vi "App - analyze RUS V6.vi"() -> ()   [LabVIEW 2015] (continued)
, "file path"=path "D:/Data/Ultrasound/LSCO/LSCO22__130814c/5_Cooling_2nd_try/September_2014/091714/50.16200K_500_2500_2.10000V_0.00000T_Sep17-2014__11-53-36_001_091714.bin", "last mod"=timestamp(3493814016 s since 1904-01-01), "file name str"="D:\\Data\\Ultrasound\\LSCO\\LSCO22__130814c\\5_Cooling_2nd_try\\September_2014\\091714\\50.16200K_500_2500_2.10000V_0.00000T_Sep17-2014__11-53-36_001_091714.bin", "mod time(min)"=58230233.6, "file format"=enum."binary", "power(V)"=2.1, "Magn Field(T) "=0.0}, {"temperature"=50.094, "temperature str"="50.09400", "file path"=path "D:/Data/Ultrasound/LSCO/LSCO22__130814c/5_Cooling_2nd_try/September_2014/091714/50.09400K_500_2500_2.10000V_0.00000T_Sep17-2014__11-54-56_001_091714.bin", "last mod"=timestamp(3493814096 s since 1904-01-01), "file name str"="D:\\Data\\Ultrasound\\LSCO\\LSCO22__130814c\\5_Cooling_2nd_try\\September_2014\\091714\\50.09400K_500_2500_2.10000V_0.00000T_Sep17-2014__11-54-56_001_091714.bin", "mod time(min)"=58230234.93333333, "file format"=enum."binary", "power(V)"=2.1, "Magn Field(T) "=0.0}, {"temperature"=50.029, "temperature str"="50.02900", "file path"=path "D:/Data/Ultrasound/LSCO/LSCO22__130814c/5_Cooling_2nd_try/September_2014/091714/50.02900K_500_2500_2.10000V_0.00000T_Sep17-2014__11-56-15_001_091714.bin", "last mod"=timestamp(3493814175 s since 1904-01-01), "file name str"="D:\\Data\\Ultrasound\\LSCO\\LSCO22__130814c\\5_Cooling_2nd_try\\September_2014\\091714\\50.02900K_500_2500_2.10000V_0.00000T_Sep17-2014__11-56-15_001_091714.bin", "mod time(min)"=58230236.25, "file format"=enum."binary", "power(V)"=2.1, "Magn Field(T) "=0.0}, {"temperature"=49.955, "temperature str"="49.95500", "file path"=path "D:/Data/Ultrasound/LSCO/LSCO22__130814c/5_Cooling_2nd_try/September_2014/091714/49.95500K_500_2500_2.10000V_0.00000T_Sep17-2014__11-57-34_001_091714.bin", "last mod"=timestamp(3493814254 s since 1904-01-01), "file name str"="D:\\Data\\Ultrasound\\LSCO\\LSCO22__130814c\\5_Cooling_2nd_try\\September_2014\\091714\\49.95500K_500_2500_2.10000V_0.00000T_Sep17-2014__11-57-34_001_091714.bin", "mod time(min)"=58230237.56666667, "file format"=enum."binary", "power(V)"=2.1, "Magn Field(T) "=0.0}, {"temperature"=49.895, "temperature str"="49.89500", "file path"=path "D:/Data/Ultrasound/LSCO/LSCO22__130814c/5_Cooling_2nd_try/September_2014/091714/49.89500K_500_2500_2.10000V_0.00000T_Sep17-2014__11-58-54_001_091714.bin", "last mod"=timestamp(3493814334 s since 1904-01-01), "file name str"="D:\\Data\\Ultrasound\\LSCO\\LSCO22__130814c\\5_Cooling_2nd_try\\September_2014\\091714\\49.89500K_500_2500_2.10000V_0.00000T_Sep17-2014__11-58-54_001_091714.bin", "mod time(min)"=58230238.9, "file format"=enum."binary", "power(V)"=2.1, "Magn Field(T) "=0.0}, {"temperature"=49.828, "temperature str"="49.82800", "file path"=path "D:/Data/Ultrasound/LSCO/LSCO22__130814c/5_Cooling_2nd_try/September_2014/091714/49.82800K_500_2500_2.10000V_0.00000T_Sep17-2014__12-00-13_001_091714.bin", "last mod"=timestamp(3493814413 s since 1904-01-01), "file name str"="D:\\Data\\Ultrasound\\LSCO\\LSCO22__130814c\\5_Cooling_2nd_try\\September_2014\\091714\\49.82800K_500_2500_2.10000V_0.00000T_Sep17-2014__12-00-13_001_091714.bin", "mod time(min)"=58230240.21666667, "file format"=enum."binary", "power(V)"=2.1, "Magn Field(T) "=0.0}, {"temperature"=49.758, "temperature str"="49.75800", "file path"=path "D:/Data/Ultrasound/LSCO/LSCO22__130814c/5_Cooling_2nd_try/September_2014/091714/49.75800K_500_2500_2.10000V_0.00000T_Sep17-2014__12-01-32_001_091714.bin", "last mod"=timestamp(3493814492 s since 1904-01-01), "file name str"="D:\\Data\\Ultrasound\\LSCO\\LSCO22__130814c\\5_Cooling_2nd_try\\September_2014\\091714\\49.75800K_500_2500_2.10000V_0.00000T_Sep17-2014__12-01-32_001_091714.bin", "mod time(min)"=58230241.53333333, "file format"=enum."binary", "power(V)"=2.1, "Magn Field(T) "=0.0}, {"temperature"=49.694, "temperature str"="49.69400", "file path"=path "D:/Data/Ultrasound/LSCO/LSCO22__130814c/5_Cooling_2nd_try/September_2014/091714/49.69400K_500_2500_2.10000V_0.00000T_Sep17-2014__12-02-52_001_091714.bin", "last mod"=timestamp(3493814572 s since 1904-01-01), "file name str"="D:\\Data\\Ultrasound\\LSCO\\LSCO22__130814c\\5_Cooling_2nd_try\\September_2014\\091714\\49.69400K_500_2500_2.10000V_0.00000T_Sep17-2014__12-02-52_001_091714.bin", "mod time(min)"=58230242.86666667, "file format"=enum."binary", "power(V)"=2.1, "Magn Field(T) "=0.0}, {"temperature"=49.627, "temperature str"="49.62700", "file path"=path "D:/Data/Ultrasound/LSCO/LSCO22__130814c/5_Cooling_2nd_try/September_2014/091714/49.62700K_500_2500_2.10000V_0.00000T_Sep17-2014__12-04-11_001_091714.bin", "last mod"=timestamp(3493814651 s since 1904-01-01), "file name str"="D:\\Data\\Ultrasound\\LSCO\\LSCO22__130814c\\5_Cooling_2nd_try\\September_2014\\091714\\49.62700K_500_2500_2.10000V_0.00000T_Sep17-2014__12-04-11_001_091714.bin", "mod time(min)"=58230244.18333333, "file format"=enum."binary", "power(V)"=2.1, "Magn Field(T) "=0.0}, {"temperature"=49.555, "temperature str"="49.55500", "file path"=path "D:/Data/Ultrasound/LSCO/LSCO22__130814c/5_Cooling_2nd_try/September_2014/091714/49.55500K_500_2500_2.10000V_0.00000T_Sep17-2014__12-05-31_001_091714.bin", "last mod"=timestamp(3493814731 s since 1904-01-01), "file name str"="D:\\Data\\Ultrasound\\LSCO\\LSCO22__130814c\\5_Cooling_2nd_try\\September_2014\\091714\\49.55500K_500_2500_2.10000V_0.00000T_Sep17-2014__12-05-31_001_091714.bin", "mod time(min)"=58230245.516666666, "file format"=enum."binary", "power(V)"=2.1, "Magn Field(T) "=0.0}, {"temperature"=49.488, "temperature str"="49.48800", "file path"=path "D:/Data/Ultrasound/LSCO/LSCO22__130814c/5_Cooling_2nd_try/September_2014/091714/49.48800K_500_2500_2.10000V_0.00000T_Sep17-2014__12-06-50_001_091714.bin", "last mod"=timestamp(3493814810 s since 1904-01-01), "file name str"="D:\\Data\\Ultrasound\\LSCO\\LSCO22__130814c\\5_Cooling_2nd_try\\September_2014\\091714\\49.48800K_500_2500_2.10000V_0.00000T_Sep17-2014__12-06-50_001_091714.bin", "mod time(min)"=58230246.833333336, "file format"=enum."binary", "power(V)"=2.1, "Magn Field(T) "=0.0}, {"temperature"=49.42, "temperature str"="49.42000", "file path"=path "D:/Data/Ultrasound/LSCO/LSCO22__130814c/5_Cooling_2nd_try/September_2014/091714/49.42000K_500_2500_2.10000V_0.00000T_Sep17-2014__12-08-09_001_091714.bin", "last mod"=timestamp(3493814889 s since 1904-01-01), "file name str"="D:\\Data\\Ultrasound\\LSCO\\LSCO22__130814c\\5_Cooling_2nd_try\\September_2014\\091714\\49.42000K_500_2500_2.10000V_0.00000T_Sep17-2014__12-08-09_001_091714.bin", "mod time(min)"=58230248.15, "file format"=enum."binary", "power(V)"=2.1, "Magn Field(T) "=0.0}, {"temperature"=49.351, "temperature str"="49.35100", "file path"=path "D:/Data/Ultrasound/LSCO/LSCO22__130814c/5_Cooling_2nd_try/September_2014/091714/49.35100K_500_2500_2.10000V_0.00000T_Sep17-2014__12-09-29_001_091714.bin", "last mod"=timestamp(3493814969 s since 1904-01-01), "file name str"="D:\\Data\\Ultrasound\\LSCO\\LSCO22__130814c\\5_Cooling_2nd_try\\September_2014\\091714\\49.35100K_500_2500_2.10000V_0.00000T_Sep17-2014__12-09-29_001_091714.bin", "mod time(min)"=58230249.483333334, "file format"=enum."binary", "power(V)"=2.1, "Magn Field(T) "=0.0}, {"temperature"=49.284, "temperature str"="49.28400", "file path"=path "D:/Data/Ultrasound/LSCO/LSCO22__130814c/5_Cooling_2nd_try/September_2014/091714/49.28400K_500_2500_2.10000V_0.00000T_Sep17-2014__12-10-48_001_091714.bin", "last mod"=timestamp(3493815048 s since 1904-01-01), "file name str"="D:\\Data\\Ultrasound\\LSCO\\LSCO22__130814c\\5_Cooling_2nd_try\\September_2014\\091714\\49.28400K_500_2500_2.10000V_0.00000T_Sep17-2014__12-10-48_001_091714.bin", "mod time(min)"=58230250.8, "file format"=enum."binary", "power(V)"=2.1, "Magn Field(T) "=0.0}, {"temperature"=49.214, "temperature str"="49.21400", "file path"=path "D:/Data/Ultrasound/LSCO/LSCO22__130814c/5_Cooling_2nd_try/September_2014/091714/49.21400K_500_2500_2.10000V_0.00000T_Sep17-2014__12-12-07_001_091714.bin", "last mod"=timestamp(3493815127 s since 1904-01-01), "file name str"="D:\\Data\\Ultrasound\\LSCO\\LSCO22__130814c\\5_Cooling_2nd_try\\September_2014\\091714\\49.21400K_500_2500_2.10000V_0.00000T_Sep17-2014__12-12-07_001_091714.bin", "mod time(min)"=58230252.11666667, "file format"=enum."binary", "power(V)"=2.1, "Magn Field(T) "=0.0}, {"temperature"=49.15, "temperature str"="49.15000", "file path"=path "D:/Data/Ultrasound/LSCO/LSCO22__130814c/5_Cooling_2nd_try/September_2014/091714/49.15000K_500_2500_2.10000V_0.00000T_Sep17-2014__12-13-27_001_091714.bin", "last mod"=timestamp(3493815207 s since 1904-01-01), "file name str"="D:\\Data\\Ultrasound\\LSCO\\LSCO22__130814c\\5_Cooling_2nd_try\\September_2014\\091714\\49.15000K_500_2500_2.10000V_0.00000T_Sep17-2014__12-13-27_001_091714.bin", "mod time(min)"=58230253.45, "file format"=enum."binary", "power(V)"=2.1, "Magn Field(T) "=0.0}, {"temperature"=49.077, "temperature str"="49.07700", "file path"=path "D:/Data/Ultrasound/LSCO/LSCO22__130814c/5_Cooling_2nd_try/September_2014/091714/49.07700K_500_2500_2.10000V_0.00000T_Sep17-2014__12-14-46_001_091714.bin", "last mod"=timestamp(3493815286 s since 1904-01-01), "file name str"="D:\\Data\\Ultrasound\\LSCO\\LSCO22__130814c\\5_Cooling_2nd_try\\September_2014\\091714\\49.07700K_500_2500_2.10000V_0.00000T_Sep17-2014__12-14-46_001_091714.bin", "mod time(min)"=58230254.766666666, "file format"=enum."binary", "power(V)"=2.1, "Magn Field(T) "=0.0}, {"temperature"=49.008, "temperature str"="49.00800", "file path"=path "D:/Data/Ultrasound/LSCO/LSCO22__130814c/5_Cooling_2nd_try/September_2014/091714/49.00800K_500_2500_2.10000V_0.00000T_Sep17-2014__12-16-06_001_091714.bin", "last mod"=timestamp(3493815366 s since 1904-01-01), "file name str"="D:\\Data\\Ultrasound\\LSCO\\LSCO22__130814c\\5_Cooling_2nd_try\\September_2014\\091714\\49.00800K_500_2500_2.10000V_0.00000T_Sep17-2014__12-16-06_001_091714.bin", "mod time(min)"=58230256.1, "file format"=enum."binary", "power(V)"=2.1, "Magn Field(T) "=0.0}, {"temperature"=48.942, "temperature str"="48.94200", "file path"=path "D:/Data/Ultrasound/LSCO/LSCO22__130814c/5_Cooling_2nd_try/September_2014/091714/48.94200K_500_2500_2.10000V_0.00000T_Sep17-2014__12-17-25_001_091714.bin", "last mod"=timestamp(3493815445 s since 1904-01-01), "file name str"="D:\\Data\\Ultrasound\\LSCO\\LSCO22__130814c\\5_Cooling_2nd_try\\September_2014\\091714\\48.94200K_500_2500_2.10000V_0.00000T_Sep17-2014__12-17-25_001_091714.bin", "mod time(min)"=58230257.416666664, "file format"=enum."binary", "power(V)"=2.1, "Magn Field(T) "=0.0}, {"temperature"=48.873, "temperature str"="48.87300", "file path"=path "D:/Data/Ultrasound/LSCO/LSCO22__130814c/5_Cooling_2nd_try/September_2014/091714/48.87300K_500_2500_2.10000V_0.00000T_Sep17-2014__12-18-44_001_091714.bin", "last mod"=timestamp(3493815524 s since 1904-01-01), "file name str"="D:\\Data\\Ultrasound\\LSCO\\LSCO22__130814c\\5_Cooling_2nd_try\\September_2014\\091714\\48.87300K_500_2500_2.10000V_0.00000T_Sep17-2014__12-18-44_001_091714.bin", "mod time(min)"=58230258.733333334, "file format"=enum."binary", "power(V)"=2.1, "Magn Field(T) "=0.0}, {"temperature"=48.805, "temperature str"="48.80500", "file path"=path "D:/Data/Ultrasound/LSCO/LSCO22__130814c/5_Cooling_2nd_try/September_2014/091714/48.80500K_500_2500_2.10000V_0.00000T_Sep17-2014__12-20-04_001_091714.bin", "last mod"=timestamp(3493815604 s since 1904-01-01), "file name str"="D:\\Data\\Ultrasound\\LSCO\\LSCO22__130814c\\5_Cooling_2nd_try\\September_2014\\091714\\48.80500K_500_2500_2.10000V_0.00000T_Sep17-2014__12-20-04_001_091714.bin", "mod time(min)"=58230260.06666667, "file format"=enum."binary", "power(V)"=2.1, "Magn Field(T) "=0.0}, {"temperature"=48.734, "temperature str"="48.73400", "file path"=path "D:/Data/Ultrasound/LSCO/LSCO22__130814c/5_Cooling_2nd_try/September_2014/091714/48.73400K_500_2500_2.10000V_0.00000T_Sep17-2014__12-21-23_001_091714.bin", "last mod"=timestamp(3493815683 s since 1904-01-01), "file name str"="D:\\Data\\Ultrasound\\LSCO\\LSCO22__130814c\\5_Cooling_2nd_try\\September_2014\\091714\\48.73400K_500_2500_2.10000V_0.00000T_Sep17-2014__12-21-23_001_091714.bin", "mod time(min)"=58230261.38333333, "file format"=enum."binary", "power(V)"=2.1, "Magn Field(T) "=0.0}, {"temperature"=48.668, "temperature str"="48.66800", "file path"=path "D:/Data/Ultrasound/LSCO/LSCO22__130814c/5_Cooling_2nd_try/September_2014/091714/48.66800K_500_2500_2.10000V_0.00000T_Sep17-2014__12-22-42_001_091714.bin", "last mod"=timestamp(3493815762 s since 1904-01-01), "file name str"="D:\\Data\\Ultrasound\\LSCO\\LSCO22__130814c\\5_Cooling_2nd_try\\September_2014\\091714\\48.66800K_500_2500_2.10000V_0.00000T_Sep17-2014__12-22-42_001_091714.bin", "mod time(min)"=58230262.7, "file format"=enum."binary", "power(V)"=2.1, "Magn Field(T) "=0.0}, {"temperature"=48.596, "temperature str"="48.59600", "file path"=path "D:/Data/Ultrasound/LSCO/LSCO22__130814c/5_Cooling_2nd_try/September_2014/091714/48.59600K_500_2500_2.10000V_0.00000T_Sep17-2014__12-24-02_001_091714.bin", "last mod"=timestamp(3493815842 s since 1904-01-01), "file name str"="D:\\Data\\Ultrasound\\LSCO\\LSCO22__130814c\\5_Cooling_2nd_try\\September_2014\\091714\\48.59600K_500_2500_2.10000V_0.00000T_Sep17-2014__12-24-02_001_091714.bin", "mod time(min)"=58230264.03333333, "file format"=enum."binary", "power(V)"=2.1, "Magn Field(T) "=0.0}, {"temperature"=48.529, "temperature str"="48.52900", "file path"=path "D:/Data/Ultrasound/LSCO/LSCO22__130814c/5_Cooling_2nd_try/September_2014/091714/48.52900K_500_2500_2.10000V_0.00000T_Sep17-2014__12-25-21_001_091714.bin", "last mod"=timestamp(3493815921 s since 1904-01-01), "file name str"="D:\\Data\\Ultrasound\\LSCO\\LSCO22__130814c\\5_Cooling_2nd_try\\September_2014\\091714\\48.52900K_500_2500_2.10000V_0.00000T_Sep17-2014__12-25-21_001_091714.bin", "mod time(min)"=58230265.35, "file format"=enum."binary", "power(V)"=2.1, "Magn Field(T) "=0.0}, {"temperature"=48.459, "temperature str"="48.45900", "file path"=path "D:/Data/Ultrasound/LSCO/LSCO22__130814c/5_Cooling_2nd_try/September_2014/091714/48.45900K_500_2500_2.10000V_0.00000T_Sep17-2014__12-26-41_001_091714.bin", "last mod"=timestamp(3493816001 s since 1904-01-01), "file name str"="D:\\Data\\Ultrasound\\LSCO\\LSCO22__130814c\\5_Cooling_2nd_try\\September_2014\\091714\\48.45900K_500_2500_2.10000V_0.00000T_Sep17-2014__12-26-41_001_091714.bin", "mod time(min)"=58230266.68333333, "file format"=enum."binary", "power(V)"=2.1, "Magn Field(T) "=0.0}, {"temperature"=48.393, "temperature str"="48.39300", "file path"=path "D:/Data/Ultrasound/LSCO/LSCO22__130814c/5_Cooling_2nd_try/September_2014/091714/48.39300K_500_2500_2.10000V_0.00000T_Sep17-2014__12-28-00_001_091714.bin", "last mod"=timestamp(3493816080 s since 1904-01-01), "file name str"="D:\\Data\\Ultrasound\\LSCO\\LSCO22__130814c\\5_Cooling_2nd_try\\September_2014\\091714\\48.39300K_500_2500_2.10000V_0.00000T_Sep17-2014__12-28-00_001_091714.bin", "mod time(min)"=58230268.0, "file format"=enum."binary", "power(V)"=2.1, "Magn Field(T) "=0.0}, {"temperature"=48.325, "temperature str"="48.32500", "file path"=path "D:/Data/Ultrasound/LSCO/LSCO22__130814c/5_Cooling_2nd_try/September_2014/091714/48.32500K_500_2500_2.10000V_0.00000T_Sep17-2014__12-29-19_001_091714.bin", "last mod"=timestamp(3493816159 s since 1904-01-01), "file name str"="D:\\Data\\Ultrasound\\LSCO\\LSCO22__130814c\\5_Cooling_2nd_try\\September_2014\\091714\\48.32500K_500_2500_2.10000V_0.00000T_Sep17-2014__12-29-19_001_091714.bin", "mod time(min)"=58230269.31666667, "file format"=enum."binary", "power(V)"=2.1, "Magn Field(T) "=0.0}, {"temperature"=48.248, "temperature str"="48.24800", "file path"=path "D:/Data/Ultrasound/LSCO/LSCO22__130814c/5_Cooling_2nd_try/September_2014/091714/48.24800K_500_2500_2.10000V_0.00000T_Sep17-2014__12-30-39_001_091714.bin", "last mod"=timestamp(3493816239 s since 1904-01-01), "file name str"="D:\\Data\\Ultrasound\\LSCO\\LSCO22__130814c\\5_Cooling_2nd_try\\September_2014\\091714\\48.24800K_500_2500_2.10000V_0.00000T_Sep17-2014__12-30-39_001_091714.bin", "mod time(min)"=58230270.65, "file format"=enum."binary", "power(V)"=2.1, "Magn Field(T) "=0.0}, {"temperature"=48.181, "temperature str"="48.18100", "file path"=path "D:/Data/Ultrasound/LSCO/LSCO22__130814c/5_Cooling_2nd_try/September_2014/091714/48.18100K_500_2500_2.10000V_0.00000T_Sep17-2014__12-31-58_001_091714.bin", "last mod"=timestamp(3493816318 s since 1904-01-01), "file name str"="D:\\Data\\Ultrasound\\LSCO\\LSCO22__130814c\\5_Cooling_2nd_try\\September_2014\\091714\\48.18100K_500_2500_2.10000V_0.00000T_Sep17-2014__12-31-58_001_091714.bin", "mod time(min)"=58230271.96666667, "file format"=enum."binary", "power(V)"=2.1, "Magn Field(T) "=0.0}, {"temperature"=48.115, "temperature str"="48.11500", "file path"=path "D:/Data/Ultrasound/LSCO/LSCO22__130814c/5_Cooling_2nd_try/September_2014/091714/48.11500K_500_2500_2.10000V_0.00000T_Sep17-2014__12-33-17_001_091714.bin", "last mod"=timestamp(3493816397 s since 1904-01-01), "file name str"="D:\\Data\\Ultrasound\\LSCO\\LSCO22__130814c\\5_Cooling_2nd_try\\September_2014\\091714\\48.11500K_500_2500_2.10000V_0.00000T_Sep17-2014__12-33-17_001_091714.bin", "mod time(min)"=58230273.28333333, "file format"=enum."binary", "power(V)"=2.1, "Magn Field(T) "=0.0}, {"temperature"=48.042, "temperature str"="48.04200", "file path"=path "D:/Data/Ultrasound/LSCO/LSCO22__130814c/5_Cooling_2nd_try/September_2014/091714/48.04200K_500_2500_2.10000V_0.00000T_Sep17-2014__12-34-37_001_091714.bin", "last mod"=timestamp(3493816477 s since 1904-01-01), "file name str"="D:\\Data\\Ultrasound\\LSCO\\LSCO22__130814c\\5_Cooling_2nd_try\\September_2014\\091714\\48.04200K_500_2500_2.10000V_0.00000T_Sep17-2014__12-34-37_001_091714.bin", "mod time(min)"=58230274.61666667, "file format"=enum."binary", "power(V)"=2.1, "Magn Field(T) "=0.0}, {"temperature"=47.973, "temperature str"="47.97300", "file path"=path "D:/Data/Ultrasound/LSCO/LSCO22__130814c/5_Cooling_2nd_try/September_2014/091714/47.97300K_500_2500_2.10000V_0.00000T_Sep17-2014__12-35-56_001_091714.bin", "last mod"=timestamp(3493816556 s since 1904-01-01), "file name str"="D:\\Data\\Ultrasound\\LSCO\\LSCO22__130814c\\5_Cooling_2nd_try\\September_2014\\091714\\47.97300K_500_2500_2.10000V_0.00000T_Sep17-2014__12-35-56_001_091714.bin", "mod time(min)"=58230275.93333333, "file format"=enum."binary", "power(V)"=2.1, "Magn Field(T) "=0.0}, {"temperature"=47.908, "temperature str"="47.90800", "file path"=path "D:/Data/Ultrasound/LSCO/LSCO22__130814c/5_Cooling_2nd_try/September_2014/091714/47.90800K_500_2500_2.10000V_0.00000T_Sep17-2014__12-37-16_001_091714.bin", "last mod"=timestamp(3493816636 s since 1904-01-01), "file name str"="D:\\Data\\Ultrasound\\LSCO\\LSCO22__130814c\\5_Cooling_2nd_try\\September_2014\\091714\\47.90800K_500_2500_2.10000V_0.00000T_Sep17-2014__12-37-16_001_091714.bin", "mod time(min)"=58230277.266666666, "file format"=enum."binary", "power(V)"=2.1, "Magn Field(T) "=0.0}, {"temperature"=47.834, "temperature str"="47.83400", "file path"=path "D:/Data/Ultrasound/LSCO/LSCO22__130814c/5_Cooling_2nd_try/September_2014/091714/47.83400K_500_2500_2.10000V_0.00000T_Sep17-2014__12-38-35_001_091714.bin", "last mod"=timestamp(3493816715 s since 1904-01-01), "file name str"="D:\\Data\\Ultrasound\\LSCO\\LSCO22__130814c\\5_Cooling_2nd_try\\September_2014\\091714\\47.83400K_500_2500_2.10000V_0.00000T_Sep17-2014__12-38-35_001_091714.bin", "mod time(min)"=58230278.583333336, "file format"=enum."binary", "power(V)"=2.1, "Magn Field(T) "=0.0}, {"temperature"=47.764, "temperature str"="47.76400", "file path"=path "D:/Data/Ultrasound/LSCO/LSCO22__130814c/5_Cooling_2nd_try/September_2014/091714/47.76400K_500_2500_2.10000V_0.00000T_Sep17-2014__12-39-54_001_091714.bin", "last mod"=timestamp(3493816794 s since 1904-01-01), "file name str"="D:\\Data\\Ultrasound\\LSCO\\LSCO22__130814c\\5_Cooling_2nd_try\\September_2014\\091714\\47.76400K_500_2500_2.10000V_0.00000T_Sep17-2014__12-39-54_001_091714.bin", "mod time(min)"=58230279.9, "file format"=enum."binary", "power(V)"=2.1, "Magn Field(T) "=0.0}, {"temperature"=47.699, "temperature str"="47.69900", "file path"=path "D:/Data/Ultrasound/LSCO/LSCO22__130814c/5_Cooling_2nd_try/September_2014/091714/47.69900K_500_2500_2.10000V_0.00000T_Sep17-2014__12-41-14_001_091714.bin", "last mod"=timestamp(3493816874 s since 1904-01-01), "file name str"="D:\\Data\\Ultrasound\\LSCO\\LSCO22__130814c\\5_Cooling_2nd_try\\September_2014\\091714\\47.69900K_500_2500_2.10000V_0.00000T_Sep17-2014__12-41-14_001_091714.bin", "mod time(min)"=58230281.233333334, "file format"=enum."binary", "power(V)"=2.1, "Magn Field(T) "=0.0}, {"temperature"=47.625, "temperature str"="47.62500", "file path"=path "D:/Data/Ultrasound/LSCO/LSCO22__130814c/5_Cooling_2nd_try/September_2014/091714/47.62500K_500_2500_2.10000V_0.00000T_Sep17-2014__12-42-33_001_091714.bin", "last mod"=timestamp(3493816953 s since 1904-01-01), "file name str"="D:\\Data\\Ultrasound\\LSCO\\LSCO22__130814c\\5_Cooling_2nd_try\\September_2014\\091714\\47.62500K_500_2500_2.10000V_0.00000T_Sep17-2014__12-42-33_001_091714.bin", "mod time(min)"=58230282.55, "file format"=enum."binary", "power(V)"=2.1, "Magn Field(T) "=0.0}, {"temperature"=47.554, "temperature str"="47.55400", "file path"=path "D:/Data/Ultrasound/LSCO/LSCO22__130814c/5_Cooling_2nd_try/September_2014/091714/47.55400K_500_2500_2.10000V_0.00000T_Sep17-2014__12-43-52_001_091714.bin", "last mod"=timestamp(3493817032 s since 1904-01-01), "file name str"="D:\\Data\\Ultrasound\\LSCO\\LSCO22__130814c\\5_Cooling_2nd_try\\September_2014\\091714\\47.55400K_500_2500_2.10000V_0.00000T_Sep17-2014__12-43-52_001_091714.bin", "mod time(min)"=58230283.86666667, "file format"=enum."binary", "power(V)"=2.1, "Magn Field(T) "=0.0}, {"temperature"=47.487, "temperature str"="47.48700", "file path"=path "D:/Data/Ultrasound/LSCO/LSCO22__130814c/5_Cooling_2nd_try/September_2014/091714/47.48700K_500_2500_2.10000V_0.00000T_Sep17-2014__12-45-12_001_091714.bin", "last mod"=timestamp(3493817112 s since 1904-01-01), "file name str"="D:\\Data\\Ultrasound\\LSCO\\LSCO22__130814c\\5_Cooling_2nd_try\\September_2014\\091714\\47.48700K_500_2500_2.10000V_0.00000T_Sep17-2014__12-45-12_001_091714.bin", "mod time(min)"=58230285.2, "file format"=enum."binary", "power(V)"=2.1, "Magn Field(T) "=0.0}, {"temperature"=47.415, "temperature str"="47.41500", "file path"=path "D:/Data/Ultrasound/LSCO/LSCO22__130814c/5_Cooling_2nd_try/September_2014/091714/47.41500K_500_2500_2.10000V_0.00000T_Sep17-2014__12-46-31_001_091714.bin", "last mod"=timestamp(3493817191 s since 1904-01-01), "file name str"="D:\\Data\\Ultrasound\\LSCO\\LSCO22__130814c\\5_Cooling_2nd_try\\September_2014\\091714\\47.41500K_500_2500_2.10000V_0.00000T_Sep17-2014__12-46-31_001_091714.bin", "mod time(min)"=58230286.516666666, "file format"=enum."binary", "power(V)"=2.1, "Magn Field(T) "=0.0}, {"temperature"=47.343, "temperature str"="47.34300", "file path"=path "D:/Data/Ultrasound/LSCO/LSCO22__130814c/5_Cooling_2nd_try/September_2014/091714/47.34300K_500_2500_2.10000V_0.00000T_Sep17-2014__12-47-51_001_091714.bin", "last mod"=timestamp(3493817271 s since 1904-01-01), "file name str"="D:\\Data\\Ultrasound\\LSCO\\LSCO22__130814c\\5_Cooling_2nd_try\\September_2014\\091714\\47.34300K_500_2500_2.10000V_0.00000T_Sep17-2014__12-47-51_001_091714.bin", "mod time(min)"=58230287.85, "file format"=enum."binary", "power(V)"=2.1, "Magn Field(T) "=0.0}, {"temperature"=47.276, "temperature str"="47.27600", "file path"=path "D:/Data/Ultrasound/LSCO/LSCO22__130814c/5_Cooling_2nd_try/September_2014/091714/47.27600K_500_2500_2.10000V_0.00000T_Sep17-2014__12-49-10_001_091714.bin", "last mod"=timestamp(3493817350 s since 1904-01-01), "file name str"="D:\\Data\\Ultrasound\\LSCO\\LSCO22__130814c\\5_Cooling_2nd_try\\September_2014\\091714\\47.27600K_500_2500_2.10000V_0.00000T_Sep17-2014__12-49-10_001_091714.bin", "mod time(min)"=58230289.166666664, "file format"=enum."binary", "power(V)"=2.1, "Magn Field(T) "=0.0}, {"temperature"=47.203, "temperature str"="47.20300", "file path"=path "D:/Data/Ultrasound/LSCO/LSCO22__130814c/5_Cooling_2nd_try/September_2014/091714/47.20300K_500_2500_2.10000V_0.00000T_Sep17-2014__12-50-29_001_091714.bin", "last mod"=timestamp(3493817429 s since 1904-01-01), "file name str"="D:\\Data\\Ultrasound\\LSCO\\LSCO22__130814c\\5_Cooling_2nd_try\\September_2014\\091714\\47.20300K_500_2500_2.10000V_0.00000T_Sep17-2014__12-50-29_001_091714.bin", "mod time(min)"=58230290.483333334, "file format"=enum."binary", "power(V)"=2.1, "Magn Field(T) "=0.0}, {"temperature"=47.135, "temperature str"="47.13500", "file path"=path "D:/Data/Ultrasound/LSCO/LSCO22__130814c/5_Cooling_2nd_try/September_2014/091714/47.13500K_500_2500_2.10000V_0.00000T_Sep17-2014__12-51-49_001_091714.bin", "last mod"=timestamp(3493817509 s since 1904-01-01), "file name str"="D:\\Data\\Ultrasound\\LSCO\\LSCO22__130814c\\5_Cooling_2nd_try\\September_2014\\091714\\47.13500K_500_2500_2.10000V_0.00000T_Sep17-2014__12-51-49_001_091714.bin", "mod time(min)"=58230291.81666667, "file format"=enum."binary", "power(V)"=2.1, "Magn Field(T) "=0.0}, {"temperature"=47.061, "temperature str"="47.06100", "file path"=path "D:/Data/Ultrasound/LSCO/LSCO22__130814c/5_Cooling_2nd_try/September_2014/091714/47.06100K_500_2500_2.10000V_0.00000T_Sep17-2014__12-53-08_001_091714.bin", "last mod"=timestamp(3493817588 s since 1904-01-01), "file name str"="D:\\Data\\Ultrasound\\LSCO\\LSCO22__130814c\\5_Cooling_2nd_try\\September_2014\\091714\\47.06100K_500_2500_2.10000V_0.00000T_Sep17-2014__12-53-08_001_091714.bin", "mod time(min)"=58230293.13333333, "file format"=enum."binary", "power(V)"=2.1, "Magn Field(T) "=0.0}, {"temperature"=46.994, "temperature str"="46.99400", "file path"=path "D:/Data/Ultrasound/LSCO/LSCO22__130814c/5_Cooling_2nd_try/September_2014/091714/46.99400K_500_2500_2.10000V_0.00000T_Sep17-2014__12-54-27_001_091714.bin", "last mod"=timestamp(3493817667 s since 1904-01-01), "file name str"="D:\\Data\\Ultrasound\\LSCO\\LSCO22__130814c\\5_Cooling_2nd_try\\September_2014\\091714\\46.99400K_500_2500_2.10000V_0.00000T_Sep17-2014__12-54-27_001_091714.bin", "mod time(min)"=58230294.45, "file format"=enum."binary", "power(V)"=2.1, "Magn Field(T) "=0.0}, {"temperature"=46.927, "temperature str"="46.92700", "file path"=path "D:/Data/Ultrasound/LSCO/LSCO22__130814c/5_Cooling_2nd_try/September_2014/091714/46.92700K_500_2500_2.10000V_0.00000T_Sep17-2014__12-55-47_001_091714.bin", "last mod"=timestamp(3493817747 s since 1904-01-01), "file name str"="D:\\Data\\Ultrasound\\LSCO\\LSCO22__130814c\\5_Cooling_2nd_try\\September_2014\\091714\\46.92700K_500_2500_2.10000V_0.00000T_Sep17-2014__12-55-47_001_091714.bin", "mod time(min)"=58230295.78333333, "file format"=enum."binary", "power(V)"=2.1, "Magn Field(T) "=0.0}, {"temperature"=46.851, "temperature str"="46.85100", "file path"=path "D:/Data/Ultrasound/LSCO/LSCO22__130814c/5_Cooling_2nd_try/September_2014/091714/46.85100K_500_2500_2.10000V_0.00000T_Sep17-2014__12-57-06_001_091714.bin", "last mod"=timestamp(3493817826 s since 1904-01-01), "file name str"="D:\\Data\\Ultrasound\\LSCO\\LSCO22__130814c\\5_Cooling_2nd_try\\September_2014\\091714\\46.85100K_500_2500_2.10000V_0.00000T_Sep17-2014__12-57-06_001_091714.bin", "mod time(min)"=58230297.1, "file format"=enum."binary", "power(V)"=2.1, "Magn Field(T) "=0.0}, {"temperature"=46.777, "temperature str"="46.77700", "file path"=path "D:/Data/Ultrasound/LSCO/LSCO22__130814c/5_Cooling_2nd_try/September_2014/091714/46.77700K_500_2500_2.10000V_0.00000T_Sep17-2014__12-58-26_001_091714.bin", "last mod"=timestamp(3493817906 s since 1904-01-01), "file name str"="D:\\Data\\Ultrasound\\LSCO\\LSCO22__130814c\\5_Cooling_2nd_try\\September_2014\\091714\\46.77700K_500_2500_2.10000V_0.00000T_Sep17-2014__12-58-26_001_091714.bin", "mod time(min)"=58230298.43333333, "file format"=enum."binary", "power(V)"=2.1, "Magn Field(T) "=0.0}, {"temperature"=46.711, "temperature str"="46.71100", "file path"=path "D:/Data/Ultrasound/LSCO/LSCO22__130814c/5_Cooling_2nd_try/September_2014/091714/46.71100K_500_2500_2.10000V_0.00000T_Sep17-2014__12-59-45_001_091714.bin", "last mod"=timestamp(3493817985 s since 1904-01-01), "file name str"="D:\\Data\\Ultrasound\\LSCO\\LSCO22__130814c\\5_Cooling_2nd_try\\September_2014\\091714\\46.71100K_500_2500_2.10000V_0.00000T_Sep17-2014__12-59-45_001_091714.bin", "mod time(min)"=58230299.75, "file format"=enum."binary", "power(V)"=2.1, "Magn Field(T) "=0.0}, {"temperature"=46.637, "temperature str"="46.63700", "file path"=path "D:/Data/Ultrasound/LSCO/LSCO22__130814c/5_Cooling_2nd_try/September_2014/091714/46.63700K_500_2500_2.10000V_0.00000T_Sep17-2014__13-01-04_001_091714.bin", "last mod"=timestamp(3493818064 s since 1904-01-01), "file name str"="D:\\Data\\Ultrasound\\LSCO\\LSCO22__130814c\\5_Cooling_2nd_try\\September_2014\\091714\\46.63700K_500_2500_2.10000V_0.00000T_Sep17-2014__13-01-04_001_091714.bin", "mod time(min)"=58230301.06666667, "file format"=enum."binary", "power(V)"=2.1, "Magn Field(T) "=0.0}, {"temperature"=46.567, "temperature str"="46.56700", "file path"=path "D:/Data/Ultrasound/LSCO/LSCO22__130814c/5_Cooling_2nd_try/September_2014/091714/46.56700K_500_2500_2.10000V_0.00000T_Sep17-2014__13-02-24_001_091714.bin", "last mod"=timestamp(3493818144 s since 1904-01-01), "file name str"="D:\\Data\\Ultrasound\\LSCO\\LSCO22__130814c\\5_Cooling_2nd_try\\September_2014\\091714\\46.56700K_500_2500_2.10000V_0.00000T_Sep17-2014__13-02-24_001_091714.bin", "mod time(min)"=58230302.4, "file format"=enum."binary", "power(V)"=2.1, "Magn Field(T) "=0.0}, {"temperature"=46.497, "temperature str"="46.49700", "file path"=path "D:/Data/Ultrasound/LSCO/LSCO22__130814c/5_Cooling_2nd_try/September_2014/091714/46.49700K_500_2500_2.10000V_0.00000T_Sep17-2014__13-03-43_001_091714.bin", "last mod"=timestamp(3493818223 s since 1904-01-01), "file name str"="D:\\Data\\Ultrasound\\LSCO\\LSCO22__130814c\\5_Cooling_2nd_try\\September_2014\\091714\\46.49700K_500_2500_2.10000V_0.00000T_Sep17-2014__13-03-43_001_091714.bin", "mod time(min)"=58230303.71666667, "file format"=enum."binary", "power(V)"=2.1, "Magn Field(T) "=0.0}, {"temperature"=46.421, "temperature str"="46.42100", "file path"=path "D:/Data/Ultrasound/LSCO/LSCO22__130814c/5_Cooling_2nd_try/September_2014/091714/46.42100K_500_2500_2.10000V_0.00000T_Sep17-2014__13-05-02_001_091714.bin", "last mod"=timestamp(3493818302 s since 1904-01-01), "file name str"="D:\\Data\\Ultrasound\\LSCO\\LSCO22__130814c\\5_Cooling_2nd_try\\September_2014\\091714\\46.42100K_500_2500_2.10000V_0.00000T_Sep17-2014__13-05-02_001_091714.bin", "mod time(min)"=58230305.03333333, "file format"=enum."binary", "power(V)"=2.1, "Magn Field(T) "=0.0}, {"temperature"=46.357, "temperature str"="46.35700", "file path"=path "D:/Data/Ultrasound/LSCO/LSCO22__130814c/5_Cooling_2nd_try/September_2014/091714/46.35700K_500_2500_2.10000V_0.00000T_Sep17-2014__13-06-22_001_091714.bin", "last mod"=timestamp(3493818382 s since 1904-01-01), "file name str"="D:\\Data\\Ultrasound\\LSCO\\LSCO22__130814c\\5_Cooling_2nd_try\\September_2014\\091714\\46.35700K_500_2500_2.10000V_0.00000T_Sep17-2014__13-06-22_001_091714.bin", "mod time(min)"=58230306.36666667, "file format"=enum."binary", "power(V)"=2.1, "Magn Field(T) "=0.0}, {"temperature"=46.279, "temperature str"="46.27900", "file path"=path "D:/Data/Ultrasound/LSCO/LSCO22__130814c/5_Cooling_2nd_try/September_2014/091714/46.27900K_500_2500_2.10000V_0.00000T_Sep17-2014__13-07-41_001_091714.bin", "last mod"=timestamp(3493818461 s since 1904-01-01), "file name str"="D:\\Data\\Ultrasound\\LSCO\\LSCO22__130814c\\5_Cooling_2nd_try\\September_2014\\091714\\46.27900K_500_2500_2.10000V_0.00000T_Sep17-2014__13-07-41_001_091714.bin", "mod time(min)"=58230307.68333333, "file format"=enum."binary", "power(V)"=2.1, "Magn Field(T) "=0.0}, {"temperature"=46.208, "temperature str"="46.20800", "file path"=path "D:/Data/Ultrasound/LSCO/LSCO22__130814c/5_Cooling_2nd_try/September_2014/091714/46.20800K_500_2500_2.10000V_0.00000T_Sep17-2014__13-09-01_001_091714.bin", "last mod"=timestamp(3493818541 s since 1904-01-01), "file name str"="D:\\Data\\Ultrasound\\LSCO\\LSCO22__130814c\\5_Cooling_2nd_try\\September_2014\\091714\\46.20800K_500_2500_2.10000V_0.00000T_Sep17-2014__13-09-01_001_091714.bin", "mod time(min)"=58230309.016666666, "file format"=enum."binary", "power(V)"=2.1, "Magn Field(T) "=0.0}, {"temperature"=46.138, "temperature str"="46.13800", "file path"=path "D:/Data/Ultrasound/LSCO/LSCO22__130814c/5_Cooling_2nd_try/September_2014/091714/46.13800K_500_2500_2.10000V_0.00000T_Sep17-2014__13-10-20_001_091714.bin", "last mod"=timestamp(3493818620 s since 1904-01-01), "file name str"="D:\\Data\\Ultrasound\\LSCO\\LSCO22__130814c\\5_Cooling_2nd_try\\September_2014\\091714\\46.13800K_500_2500_2.10000V_0.00000T_Sep17-2014__13-10-20_001_091714.bin", "mod time(min)"=58230310.333333336, "file format"=enum."binary", "power(V)"=2.1, "Magn Field(T) "=0.0}, {"temperature"=46.066, "temperature str"="46.06600", "file path"=path "D:/Data/Ultrasound/LSCO/LSCO22__130814c/5_Cooling_2nd_try/September_2014/091714/46.06600K_500_2500_2.10000V_0.00000T_Sep17-2014__13-11-39_001_091714.bin", "last mod"=timestamp(3493818699 s since 1904-01-01), "file name str"="D:\\Data\\Ultrasound\\LSCO\\LSCO22__130814c\\5_Cooling_2nd_try\\September_2014\\091714\\46.06600K_500_2500_2.10000V_0.00000T_Sep17-2014__13-11-39_001_091714.bin", "mod time(min)"=58230311.65, "file format"=enum."binary", "power(V)"=2.1, "Magn Field(T) "=0.0}, {"temperature"=45.994, "temperature str"="45.99400", "file path"=path "D:/Data/Ultrasound/LSCO/LSCO22__130814c/5_Cooling_2nd_try/September_2014/091714/45.99400K_500_2500_2.10000V_0.00000T_Sep17-2014__13-12-59_001_091714.bin", "last mod"=timestamp(3493818779 s since 1904-01-01), "file name str"="D:\\Data\\Ultrasound\\LSCO\\LSCO22__130814c\\5_Cooling_2nd_try\\September_2014\\091714\\45.99400K_500_2500_2.10000V_0.00000T_Sep17-2014__13-12-59_001_091714.bin", "mod time(min)"=58230312.983333334, "file format"=enum."binary", "power(V)"=2.1, "Magn Field(T) "=0.0}, {"temperature"=45.923, "temperature str"="45.92300", "file path"=path "D:/Data/Ultrasound/LSCO/LSCO22__130814c/5_Cooling_2nd_try/September_2014/091714/45.92300K_500_2500_2.10000V_0.00000T_Sep17-2014__13-14-18_001_091714.bin", "last mod"=timestamp(3493818858 s since 1904-01-01), "file name str"="D:\\Data\\Ultrasound\\LSCO\\LSCO22__130814c\\5_Cooling_2nd_try\\September_2014\\091714\\45.92300K_500_2500_2.10000V_0.00000T_Sep17-2014__13-14-18_001_091714.bin", "mod time(min)"=58230314.3, "file format"=enum."binary", "power(V)"=2.1, "Magn Field(T) "=0.0}, {"temperature"=45.848, "temperature str"="45.84800", "file path"=path "D:/Data/Ultrasound/LSCO/LSCO22__130814c/5_Cooling_2nd_try/September_2014/091714/45.84800K_500_2500_2.10000V_0.00000T_Sep17-2014__13-15-37_001_091714.bin", "last mod"=timestamp(3493818937 s since 1904-01-01), "file name str"="D:\\Data\\Ultrasound\\LSCO\\LSCO22__130814c\\5_Cooling_2nd_try\\September_2014\\091714\\45.84800K_500_2500_2.10000V_0.00000T_Sep17-2014__13-15-37_001_091714.bin", "mod time(min)"=58230315.61666667, "file format"=enum."binary", "power(V)"=2.1, "Magn Field(T) "=0.0}, {"temperature"=45.779, "temperature str"="45.77900", "file path"=path "D:/Data/Ultrasound/LSCO/LSCO22__130814c/5_Cooling_2nd_try/September_2014/091714/45.77900K_500_2500_2.10000V_0.00000T_Sep17-2014__13-16-57_001_091714.bin", "last mod"=timestamp(3493819017 s since 1904-01-01), "file name str"="D:\\Data\\Ultrasound\\LSCO\\LSCO22__130814c\\5_Cooling_2nd_try\\September_2014\\091714\\45.77900K_500_2500_2.10000V_0.00000T_Sep17-2014__13-16-57_001_091714.bin", "mod time(min)"=58230316.95, "file format"=enum."binary", "power(V)"=2.1, "Magn Field(T) "=0.0}, {"temperature"=45.704, "temperature str"="45.70400", "file path"=path "D:/Data/Ultrasound/LSCO/LSCO22__130814c/5_Cooling_2nd_try/September_2014/091714/45.70400K_500_2500_2.10000V_0.00000T_Sep17-2014__13-18-16_001_091714.bin", "last mod"=timestamp(3493819096 s since 1904-01-01), "file name str"="D:\\Data\\Ultrasound\\LSCO\\LSCO22__130814c\\5_Cooling_2nd_try\\September_2014\\091714\\45.70400K_500_2500_2.10000V_0.00000T_Sep17-2014__13-18-16_001_091714.bin", "mod time(min)"=58230318.266666666, "file format"=enum."binary", "power(V)"=2.1, "Magn Field(T) "=0.0}, {"temperature"=45.63, "temperature str"="45.63000", "file path"=path "D:/Data/Ultrasound/LSCO/LSCO22__130814c/5_Cooling_2nd_try/September_2014/091714/45.63000K_500_2500_2.10000V_0.00000T_Sep17-2014__13-19-36_001_091714.bin", "last mod"=timestamp(3493819176 s since 1904-01-01), "file name str"="D:\\Data\\Ultrasound\\LSCO\\LSCO22__130814c\\5_Cooling_2nd_try\\September_2014\\091714\\45.63000K_500_2500_2.10000V_0.00000T_Sep17-2014__13-19-36_001_091714.bin", "mod time(min)"=58230319.6, "file format"=enum."binary", "power(V)"=2.1, "Magn Field(T) "=0.0}, {"temperature"=45.56, "temperature str"="45.56000", "file path"=path "D:/Data/Ultrasound/LSCO/LSCO22__130814c/5_Cooling_2nd_try/September_2014/091714/45.56000K_500_2500_2.10000V_0.00000T_Sep17-2014__13-20-55_001_091714.bin", "last mod"=timestamp(3493819255 s since 1904-01-01), "file name str"="D:\\Data\\Ultrasound\\LSCO\\LSCO22__130814c\\5_Cooling_2nd_try\\September_2014\\091714\\45.56000K_500_2500_2.10000V_0.00000T_Sep17-2014__13-20-55_001_091714.bin", "mod time(min)"=58230320.916666664, "file format"=enum."binary", "power(V)"=2.1, "Magn Field(T) "=0.0}, {"temperature"=45.483, "temperature str"="45.48300", "file path"=path "D:/Data/Ultrasound/LSCO/LSCO22__130814c/5_Cooling_2nd_try/September_2014/091714/45.48300K_500_2500_2.10000V_0.00000T_Sep17-2014__13-22-14_001_091714.bin", "last mod"=timestamp(3493819334 s since 1904-01-01), "file name str"="D:\\Data\\Ultrasound\\LSCO\\LSCO22__130814c\\5_Cooling_2nd_try\\September_2014\\091714\\45.48300K_500_2500_2.10000V_0.00000T_Sep17-2014__13-22-14_001_091714.bin", "mod time(min)"=58230322.233333334, "file format"=enum."binary", "power(V)"=2.1, "Magn Field(T) "=0.0}, {"temperature"=45.412, "temperature str"="45.41200", "file path"=path "D:/Data/Ultrasound/LSCO/LSCO22__130814c/5_Cooling_2nd_try/September_2014/091714/45.41200K_500_2500_2.10000V_0.00000T_Sep17-2014__13-23-34_001_091714.bin", "last mod"=timestamp(3493819414 s since 1904-01-01), "file name str"="D:\\Data\\Ultrasound\\LSCO\\LSCO22__130814c\\5_Cooling_2nd_try\\September_2014\\091714\\45.41200K_500_2500_2.10000V_0.00000T_Sep17-2014__13-23-34_001_091714.bin", "mod time(min)"=58230323.56666667, "file format"=enum."binary", "power(V)"=2.1, "Magn Field(T) "=0.0}, {"temperature"=45.339, "temperature str"="45.33900", "file path"=path "D:/Data/Ultrasound/LSCO/LSCO22__130814c/5_Cooling_2nd_try/September_2014/091714/45.33900K_500_2500_2.10000V_0.00000T_Sep17-2014__13-24-53_001_091714.bin", "last mod"=timestamp(3493819493 s since 1904-01-01), "file name str"="D:\\Data\\Ultrasound\\LSCO\\LSCO22__130814c\\5_Cooling_2nd_try\\September_2014\\091714\\45.33900K_500_2500_2.10000V_0.00000T_Sep17-2014__13-24-53_001_091714.bin", "mod time(min)"=58230324.88333333, "file format"=enum."binary", "power(V)"=2.1, "Magn Field(T) "=0.0}, {"temperature"=45.268, "temperature str"="45.26800", "file path"=path "D:/Data/Ultrasound/LSCO/LSCO22__130814c/5_Cooling_2nd_try/September_2014/091714/45.26800K_500_2500_2.10000V_0.00000T_Sep17-2014__13-26-12_001_091714.bin", "last mod"=timestamp(3493819572 s since 1904-01-01), "file name str"="D:\\Data\\Ultrasound\\LSCO\\LSCO22__130814c\\5_Cooling_2nd_try\\September_2014\\091714\\45.26800K_500_2500_2.10000V_0.00000T_Sep17-2014__13-26-12_001_091714.bin", "mod time(min)"=58230326.2, "file format"=enum."binary", "power(V)"=2.1, "Magn Field(T) "=0.0}, {"temperature"=45.196, "temperature str"="45.19600", "file path"=path "D:/Data/Ultrasound/LSCO/LSCO22__130814c/5_Cooling_2nd_try/September_2014/091714/45.19600K_500_2500_2.10000V_0.00000T_Sep17-2014__13-27-32_001_091714.bin", "last mod"=timestamp(3493819652 s since 1904-01-01), "file name str"="D:\\Data\\Ultrasound\\LSCO\\LSCO22__130814c\\5_Cooling_2nd_try\\Sept
